vi "rearrengeArray.vi"(0 "array in":dbl[](array[numeric]), 1 "desired size":u16) -> (2 "array out":dbl[](array[numeric]))   [LabVIEW 2023]
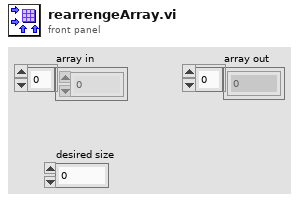
[diagram p1: front panel]
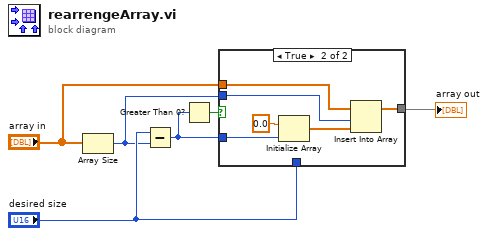
[diagram p0: block diagram]
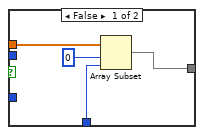
[diagram p2: hidden frame]
diagram:
  n1 = Array Size(array="array in") -> (size(s)=w1:i32)
  n2 = Subtract(x="desired size", y=w1) -> (x-y=w6:i32)
  n3 = Greater Than 0?(x=w6) -> (x > 0?=w5:bool)
  n4 = case shown="True" w5 {
    tunnel: "array in" -> [w10 w15]
    tunnel: [w9 w13] -> w3
    tunnel: "desired size" -> [w7 _]
    tunnel: w6 -> [_ w12]
    tunnel: w1 -> [_ w11]
    frame False {
      n5 = Array Subset(array=w10, index=0, length=w7) -> (w9:dbl[])
    }
    frame True {
      n6 = Initialize Array(0.0 ("element"), w12) -> (w14:dbl[])
      n7 = Insert Into Array(array=w15, index=w11, new element=w14) -> (w13:dbl[])
    }
  }
  "array out" <- w3
